vi "SetExternalInterfaces.vi"(8 "ErrorIn":errorcluster, 10 "ExternalInterfaces":T1[](array[typedef]), 11 "ReferenceIn":refnum<class "BusBase.lvclass">) -> (0 "ErrorOut":errorcluster, 3 "ReferenceOut":refnum<class "BusBase.lvclass">)   [LabVIEW 2021, in "BusBase.lvlib" / "BusBase.lvclass"]
doc: "Sets the external interface objects that are used by the object. Each interface is defined by:\n\n- the label of the control in the attribute cluster of the object\n\n- the object inself that inherits from the attribute control\n\n- a boolean that indicates if this an array of objects"
uses:
  BusBase.lvclass
  Library_TAF_Support/ClusterArrayConversion/BundledArray.ctl
  ae6ad4b9-ae21-447e-8e47-b28872e81ddf.vi
  <userlib>/_OpenG.lib/lvdata/lvdata.llb/Get Cluster Element Names__ogtk.vi
  Library_TAF_Support/ClusterArrayConversion/ClusterArrayConversion.lvlib
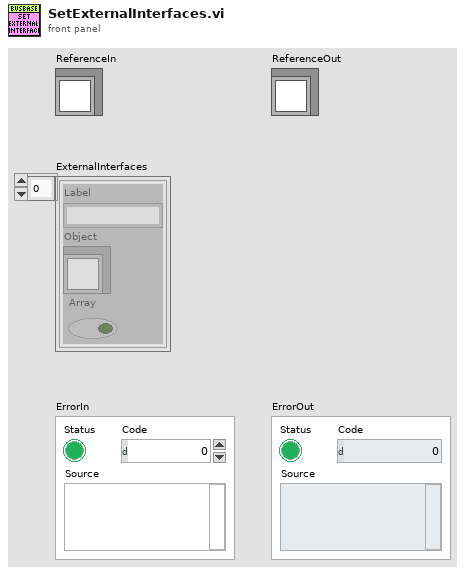
[diagram p1: front panel]
types:
  T1 = typedef "ClusterArrayConversion.lvlib/BundledArray.ctl" = cluster{"Label":string, "Object":refnum<class>, "Array":bool}
  T2 = typedef "BusBase.lvlib/BusBase.lvclass/ObjectAttributes.ctl" = cluster{"Interfaces":cluster{"TargetClasses":refnum<class>[]}, "Locals":cluster{"MainGUIActive":refnum<queue>}, "Persistent":cluster{"Dummy":bool}}
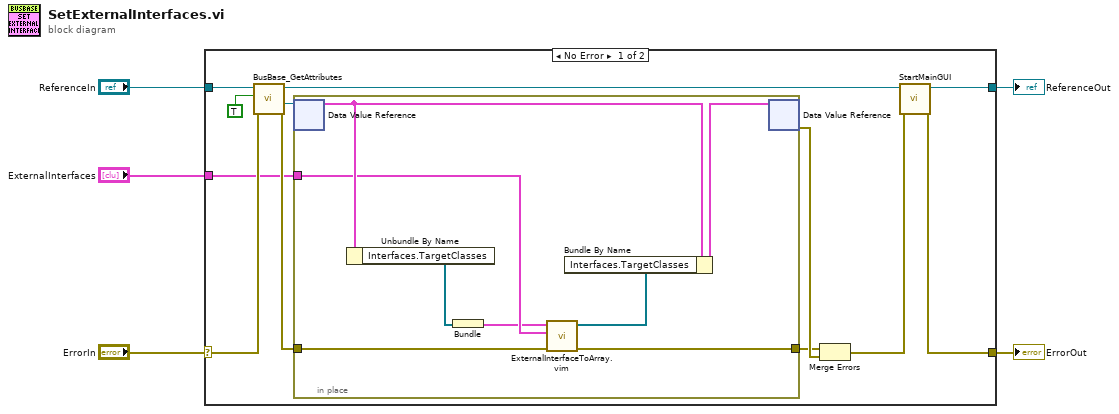
[diagram p0: block diagram]
diagram:
  n1 = case shown="No Error" "ErrorIn" {
    selector: "ErrorIn" -> [w17 w27]
    tunnel: [w12 w27] -> w4
    tunnel: [w6 w26] -> w2
    tunnel: "ReferenceIn" -> [w11 w26]
    tunnel: "ExternalInterfaces" -> [w7 _]
    frame No Error {
      n2 = call "BusBase_GetAttributes.vi"("ErrorIn"=w17, "OnlyGetDvrReference(False)"=TRUE, "ReferenceIn"=w11) -> ("ErrorOut"=w14:errorcluster, "DataRef"=w8:refnum<data-value>, "ReferenceOut"=w10:refnum<class "BusBase.lvclass">)  [unwired: 5 in, 1 out]
      n3 = in-place {
        in-place-border: [w24] -> w15
        in-place-border: w14 -> [w25]
        in-place-border: w7 -> [w21]
        n4 = in-place-dvr #1(w8) -> (w22:T2)  [unwired: 1 out]
        n5 = Unbundle By Name(w22) -> ("Interfaces.TargetClasses"=w19:refnum<class>[])
        n6 = Bundle("TargetClasses"=w19) -> (w18:cluster{"TargetClasses":refnum<class>[]})  [unwired: 1 in]
        n7 = call "ExternalInterfaceToArray.vim"("ErrorIn"=w25, "ExternalInterfaces"=w21, "TypeIn"=w18) -> ("ErrorOut"=w24:errorcluster, "ArrayOut"=w20:refnum<class>[])  [unwired: 7 in]
        n8 = Bundle By Name(cluster=w22, "Interfaces.TargetClasses"=w20) -> (w23:T2)
        n9 = in-place-dvr #1(w23) -> (w16:errorcluster)  [unwired: 1 out]
      }
      n10 = Merge Errors(w15, w16) -> (w13:errorcluster)
      n11 = call "StartMainGUI.vi"("ErrorIn"=w13, "ReferenceIn"=w10) -> ("ErrorOut"=w12:errorcluster, "ReferenceOut"=w6:refnum<class "BusBase.lvclass">)  [unwired: 6 in, 2 out]
    }
    frame Error {
    }
  }
  "ErrorOut" <- w4
  "ReferenceOut" <- w2
